vi "5.7-Any_UDP_Client.vi"(7 "Port In":refnum<k16>, 8 "error In":errorcluster, 9 "Max Size":i32, 11 "DataTypeIn":variant) -> (0 "Error Out":errorcluster, 2 "Check Passed":bool, 3 "DataOut":variant, 5 "Port out":refnum<k16>)   [LabVIEW 2010]
doc: "Runs a simple UDP Client which sends a five charactor hello before awaiting a responce. This function has timeouts which guarentee that it finishes, but do not guarentee that it received data. Check Passed tells you if the data is good (if there is an error it defaults to false)."
panel:
  out "Rawdata out":string
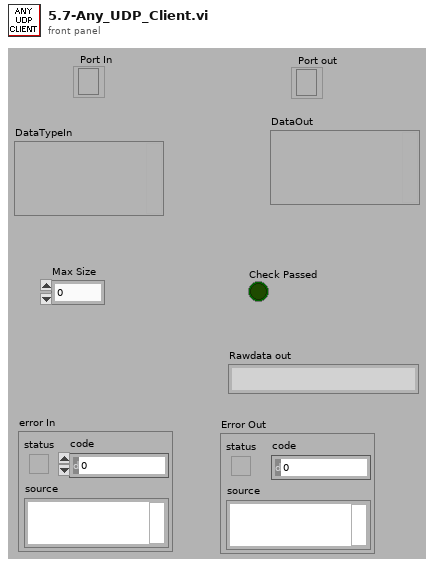
[diagram p1: front panel]
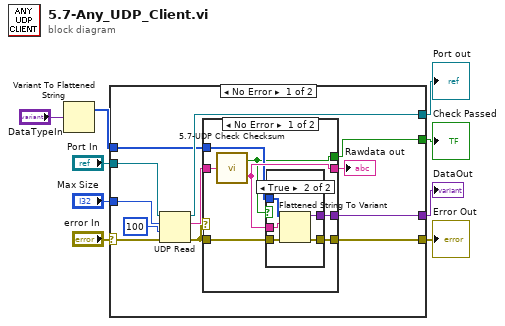
[diagram p0: block diagram]
diagram:
  n1 = Variant To Flattened String(Variant="DataTypeIn") -> (1:w8:i16[])  [unwired: 1 out]
  n2 = case shown="No Error" "error In" {
    selector: "error In" -> [w21 w37]
    tunnel: "Port In" -> [w20 w38]
    tunnel: [w19 w38] -> w7
    tunnel: [w12 w37] -> w6
    tunnel: w8 -> [w14 _]
    tunnel: [w15 _] -> w3
    tunnel: [w11 _] -> w2
    tunnel: "Max Size" -> [w10 _]
    frame No Error {
      n3 = UDP Read(connection ID=w20, max size (548)=w10, timeout ms (25000)=100, 8:w21) -> (data out=w17:string, error out=w13:errorcluster, 3:w19:refnum<k16>)  [unwired: 2 out]
      n4 = case shown="No Error" w13 {
        tunnel: w17 -> [w28 w36]
        tunnel: [w27 w36] -> w16
        tunnel: [w22 _] -> w15
        tunnel: w14 -> [w26 _]
        tunnel: w13 -> [w25 w35]
        tunnel: [w24 w35] -> w12
        tunnel: [w23 _] -> w11
        frame No Error {
          n5 = call "5.7-UDP Check Checksum.vi"("CS string in"=w28) -> ("CS string in 2"=w27:string, "Boolean"=w22:bool)
          n6 = case shown="True" w22 {
            tunnel: w27 -> [_ w34]
            tunnel: w26 -> [_ w33]
            tunnel: w25 -> [w29 w32]
            tunnel: [w29 w31] -> w24
            tunnel: [_ w30] -> w23
            frame False {
            }
            frame True {
              n7 = Flattened String To Variant(4:w32, 6:w34, 7:w33) -> (0:w31:errorcluster, 3:w30:variant)
            }
          }
        }
        frame Error {
        }
      }
      "Rawdata out" <- w16
    }
    frame Error {
    }
  }
  "DataOut" <- w2
  "Port out" <- w7
  "Error Out" <- w6
  "Check Passed" <- w3
